vi "HV_Import_Status_from_sethv.vi"() -> (0 "output array":string[][](array[string]), 2 "Error":string, 3 "transposed array":string[][](array[string]))   [LabVIEW 2018]
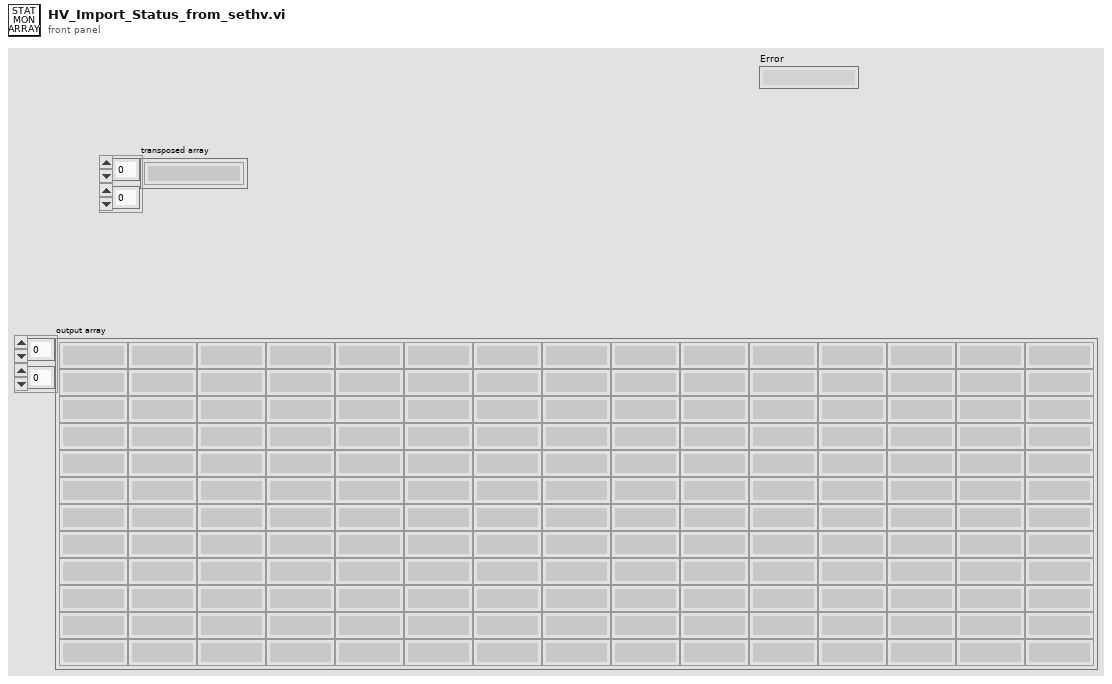
[diagram p1: front panel]
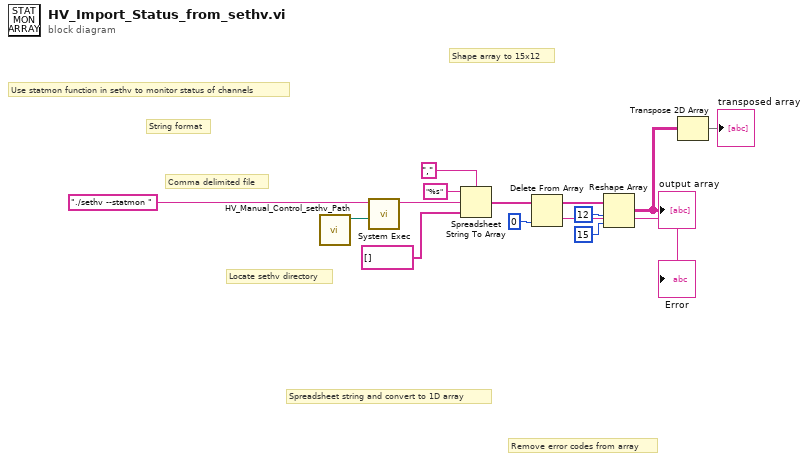
[diagram p0: block diagram]
diagram:
  # "Locate sethv directory"
  # "String format"
  # "Comma delimited file"
  # "Shape array to 15x12"
  # "Remove error codes from array"
  # "Spreadsheet string and convert to 1D array"
  # "Use statmon function in sethv to monitor status of channels"
  n1 = call "HV_Manual_Control_sethv_Path.vi"() -> ("sethv filepath"=w14:path)  [unwired: 11 in]
  n2 = call <vilib>:"System Exec.vi"("working directory"=w14, "command line"="./sethv --statmon " ("string")) -> ("standard output"=w4:string)  [unwired: 6 in, 3 out]
  n3 = Spreadsheet String To Array(delimiter (Tab)=",", format string="%s", spreadsheet string=w4, array type (2D Dbl)=string[] []) -> (array=w8:string[])
  n4 = Delete From Array(array=w8, index=0) -> (deleted portion=→"Error":string, array with subset deleted=w10:string[])  [unwired: 1 in]
  n5 = Reshape Array(w10, 12 ("dimension size"), 15 ("dimension size")) -> (w13:string[][])
  "output array" <- w13
  n6 = Transpose 2D Array(2D array=w13) -> (transposed array=→"transposed array":string[][])
